vi "StringAsValue.vi"(8 "error in":errorcluster, 11 "scalar value (string)":string) -> (0 "error out":errorcluster, 3 "scalar string":string)   [LabVIEW 2014]
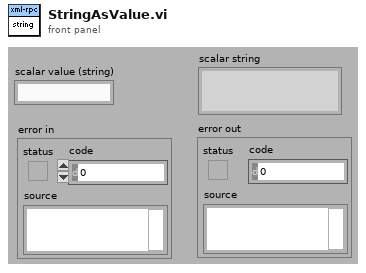
[diagram p1: front panel]
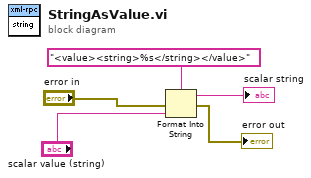
[diagram p0: block diagram]
diagram:
  n1 = Format Into String(format string="<value><string>%s</string></value>", error in="error in", "scalar value (string)") -> (resulting string=→"scalar string":string, error out=→"error out":errorcluster)  [unwired: 1 in]
